vi "Build Tags.vi"(8 "error in (no error)":errorcluster, 11 "USB DAQ in":refnum<class "USB DAQ.lvclass">) -> (0 "error out":errorcluster, 3 "USB DAQ out":refnum<class "USB DAQ.lvclass">)   [LabVIEW 2025, in "USB DAQ.lvclass"]
uses:
  USB DAQ.lvclass
  USB DAQ.lvclass/USB DAQ.ctl
  ae97a586-9584-4722-9bcd-738e0a7806d0.vi
  381b6728-7cba-47ee-b600-8bd233dc363b.vi
  a1829b52-977b-4372-a9b5-10549a913770.vi
panel:
  # "This VI is called by Pre-Launch Init"
  # "Handler's Tags should be created here"
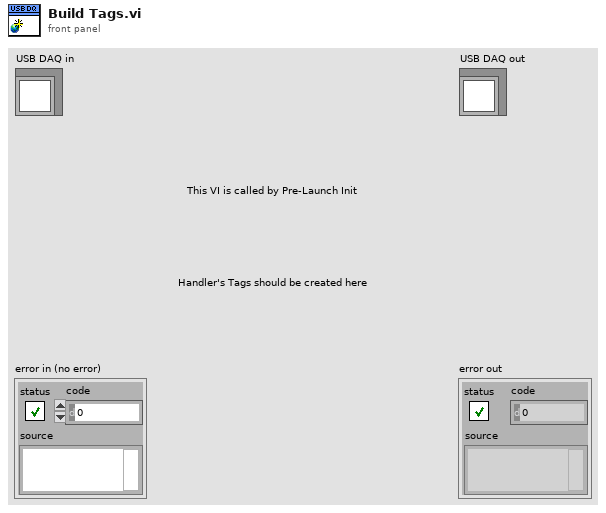
[diagram p1: front panel]
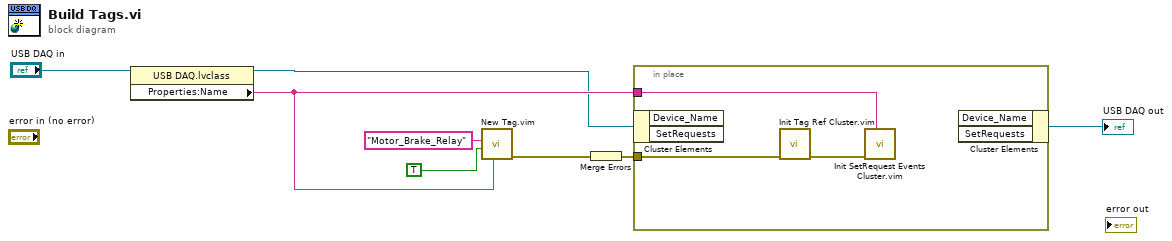
[diagram p0: block diagram]
diagram:
  n1 = property class="USB DAQ.lvclass"(reference="USB DAQ in") -> (reference out=w2:refnum<class "USB DAQ.lvclass">, "Properties:Name"=w3:string)  [unwired: 1 in, 1 out]
  n2 = call "New Tag.vim"("Namespace"=w3, "Initial Value"=TRUE, "Tag Name"="Motor_Brake_Relay") -> ("error out"=w5:errorcluster)  [unwired: 7 in, 1 out]
  n3 = Merge Errors(w5) -> (w4:errorcluster)
  n4 = in-place {
    in-place-border: w4 -> [w11]
    in-place-border: w3 -> [w10]
    n5 = in-place-cluster #1(w2) -> ()  [unwired: 2 out]
    n6 = call "Init Tag Ref Cluster.vim"("error in (no error)"=w11) -> ("error out"=w9:errorcluster)  [unwired: 8 in, 2 out]
    n7 = call "Init SetRequest Events Cluster.vim"("Namespace"=w10, "error in (no error)"=w9) -> ()  [unwired: 8 in, 2 out]
    n8 = in-place-cluster #1() -> (→"USB DAQ out":refnum<class "USB DAQ.lvclass">)  [unwired: 2 in]
  }
